vi "Sequence.vi"(7 "Name":string="Sequence", 11 "Nodes":refnum<class "abs_Node.lvclass">[](array[class])) -> (3 "Node":refnum<class "abs_Node.lvclass">)   [LabVIEW 2021, in "BT.lvlib"]
uses:
  BT.lvlib
  abs_Node/abs_Node.lvclass
  Sequence/Sequence.lvclass
  C:/Users/Tim/Documents/LabVIEW/2021/Behaviour Tree/Source/abs_Composite/abs_Composite.lvclass
  C:/Users/Tim/Documents/LabVIEW/2021/Behaviour Tree/Source/abs_Node/abs_Node.lvclass
  abs_Composite/abs_Composite.lvclass/abs_Composite.ctl
  abs_Node/abs_Node.lvclass/abs_Node.ctl
  abs_Composite/Properties/Write Nodes.vi
  abs_Node/Properties/Write Name.vi
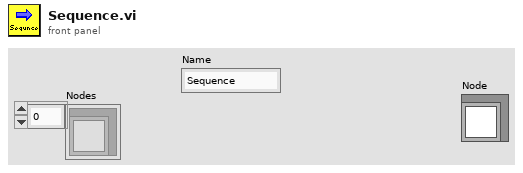
[diagram p1: front panel]
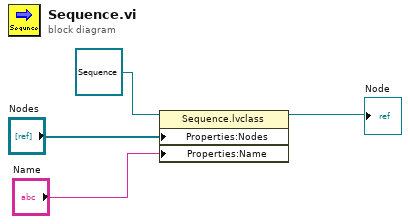
[diagram p0: block diagram]
diagram:
  n1 = property class="Sequence.lvclass"(reference=refnum<class "Sequence.lvclass"> refnum ("BT.lvlib:Sequence.lvclass"), "Properties:Nodes"="Nodes", "Properties:Name"="Name") -> (reference out=→"Node":refnum<class "Sequence.lvclass">)  [unwired: 1 in, 1 out]
